vi "wait_for_movement.vi"(8 "error in (no error)":errorcluster, 11 "IScan in":refnum<k7>) -> (0 "error out":errorcluster, 3 "IScan out":refnum<k7>)   [LabVIEW 2011]
uses:
  stage_modules/Globals.vi
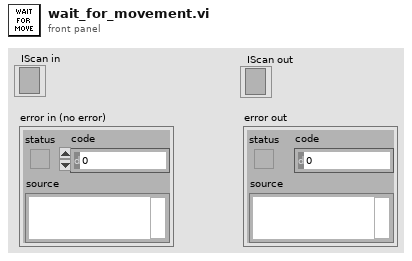
[diagram p1: front panel]
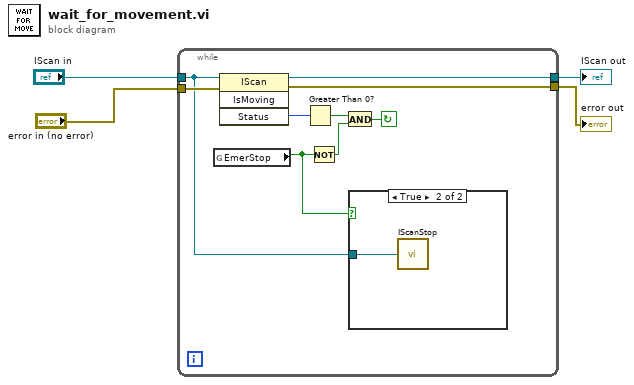
[diagram p0: block diagram]
diagram:
  n1 = while {
    tunnel: "IScan in" -> [w7]
    tunnel: "error in (no error)" -> [w9]
    tunnel: [w6] -> w2
    tunnel: [w5] -> w1
    stop <- w11 continue-if-true
    n2 = global read "Globals.vi" "EmerStop"() -> (w8:bool)
    n3 = invoke class="IScan" method="IsMoving"(reference=w7, error in=w9) -> (reference out=w5:refnum<k7>, error out=w6:errorcluster, "Status"=w10:i32)  [unwired: 2 in, 1 out]
    n4 = Greater Than 0?(x=w10) -> (x > 0?=w13:bool)
    n5 = Not(x=w8) -> (.not. x?=w12:bool)
    n6 = And(x=w13, y=w12) -> (x .and. y?=w11:bool)
    n7 = case shown="True" w8 {
      tunnel: w7 -> [_ w14]
      frame False {
      }
      frame True {
        n8 = call "IScanStop.vi"("PRIORLib.IScanIn"=w14) -> ()  [unwired: 3 out]
      }
    }
  }
  "error out" <- w2
  "IScan out" <- w1
